vi "Stoerungen (1-64) - Anlagengrenzw..vi"(8 "Fehler (Eingang)":errorcluster caption="Fehler (Eingang, kein Fehler)") -> (0 "Fehler (Ausgang)":errorcluster)   [LabVIEW 2020, in "Stoermeldungen.lvlib"]
uses:
  Stoermeldungen.lvlib
  Stoerungen 1-64.ctl
  Seiten/Anlagengrenzwerte/Anlagen-Parameternamen.ctl
  Aktion Heizung Uebertemperatur.ctl
  Verwaltung/FGV IN Aktionen.ctl
  FGV Stoerungen Aktionen.ctl
  Aktion Anlagengrenzen pruefen.ctl
  Seiten/Anlagengrenzwerte/Anlagengrenzwerte.lvlib
  Verwaltung/Verwaltung - cRIO.lvlib
panel:
  # "Störmeldungen:\n\nAnlagengrenzwerte (1-64)"
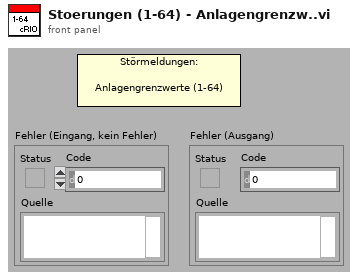
[diagram p1: front panel]
types:
  T1 = typedef "Anlagengrenzwerte.lvlib/Anlagen-Parameternamen.ctl" = enum16{"Eingangsdruck FT-IR:", "Durchfluss FT-IR:", "Durchfluss CalGas", "Druck Ausgang", "Druck Kalter Block", "Heizleitung intern", "Heizleitung zu FT-IR", "Heizung Filter:", "Heizung Pumpe:", "HL Extern SP1", "HL Extern SP2", "FT-IR Messzelle", "Schaltschrank", "Gaskühler"}
  T2 = typedef "Stoermeldungen.lvlib/FGV Stoerungen Aktionen.ctl" = enum16{"lesen", "Störung aktiv?", "1-64", "65-128"}
  T3 = typedef "Verwaltung - cRIO.lvlib/FGV IN Aktionen.ctl" = enum16{"lesen", "DI", "AI", "Fühler Br.", "TC", "Fühler Br. TC"}
  T4 = typedef "Stoermeldungen.lvlib/Aktion Heizung Uebertemperatur.ctl" = enum16{"lesen", "prüfen", "rücksetzen"}
  T5 = typedef "Stoermeldungen.lvlib/Stoerungen 1-64.ctl" = cluster{"ERR. 1":bool, "ERR. 2":bool, "ERR. 3":bool, "ERR. 4":bool, "ERR. 5":bool, "ERR. 6":bool, "ERR. 7":bool, "ERR. 8":bool, "ERR. 9":bool, "ERR. 10":bool, "ERR. 11":bool, "ERR. 12":bool, "ERR. 13":bool, "ERR. 14":bool, "ERR. 15":bool, "ERR. 16":bool, "ERR. 17":bool, "ERR. 18":bool, "ERR. 19":bool, "ERR. 20":bool, "ERR. 21":bool, "ERR. 22":bool, "ERR. 23":bool, "ERR. 24":bool, "ERR. 25":bool, "ERR. 26":bool, "ERR. 27":bool, "ERR. 28":bool, "ERR. 29":bool, "ERR. 30":bool, "ERR. 31":bool, "ERR. 32":bool, "ERR. 33":bool, "ERR. 34":bool, "ERR. 35":bool, "ERR. 36":bool, "ERR. 37":bool, "ERR. 38":bool, "ERR. 39":bool, "ERR. 40":bool, "ERR. 41":bool, "ERR. 42":bool, "ERR. 43":bool, "ERR. 44":bool, "ERR. 45":bool, "ERR. 46":bool, "ERR. 47":bool, "ERR. 48":bool, "ERR. 49":bool, "ERR. 50":bool, "ERR. 51":bool, "ERR. 52":bool, "ERR. 53":bool, "ERR. 54":bool, "ERR. 55":bool, "ERR. 56":bool, "ERR. 57":bool, "ERR. 58":bool, "ERR. 59":bool, "ERR. 60":bool, "ERR. 61":bool, "ERR. 62":bool, "ERR. 63":bool, "ERR. 64":bool}
  T6 = typedef "Verwaltung - cRIO.lvlib/TC Eingaenge.ctl" = cluster{"TC0: Reserve":sgl, "TC1: HL zu FT-IR":sgl, "TC2: HL Extern SP1":sgl, "TC3: HL Extern SP2":sgl, "TC4: Reserve":sgl, "TC5: Reserve":sgl, "TC6: Reserve":sgl, "TC7: Reserve":sgl, "TC8: FT-IR":sgl, "TC9: Reserve":sgl, "TC10: Schaltschrank":sgl, "TC11: Umgebung":sgl}
  T7 = typedef "Stoermeldungen.lvlib/Aktion Anlagengrenzen pruefen.ctl" = enum16{"Temp.", "HKL", "Druck", "SS Temp."}
  T8 = typedef "Anlagengrenzwerte.lvlib/Anlagen-Parameternamen.ctl" = enum16{"Eingangsdruck FT-IR:", "Durchfluss FT-IR:", "Druck Ausgang", "Druck Kalter Block", "Heizleitung intern", "Heizung Filter:", "Heizung Pumpe:", "HL Extern SP1", "HL Extern SP2", "FT-IR Messzelle", "Schaltschrank", "Gaskühler", "Reserve", "Flussregler"}
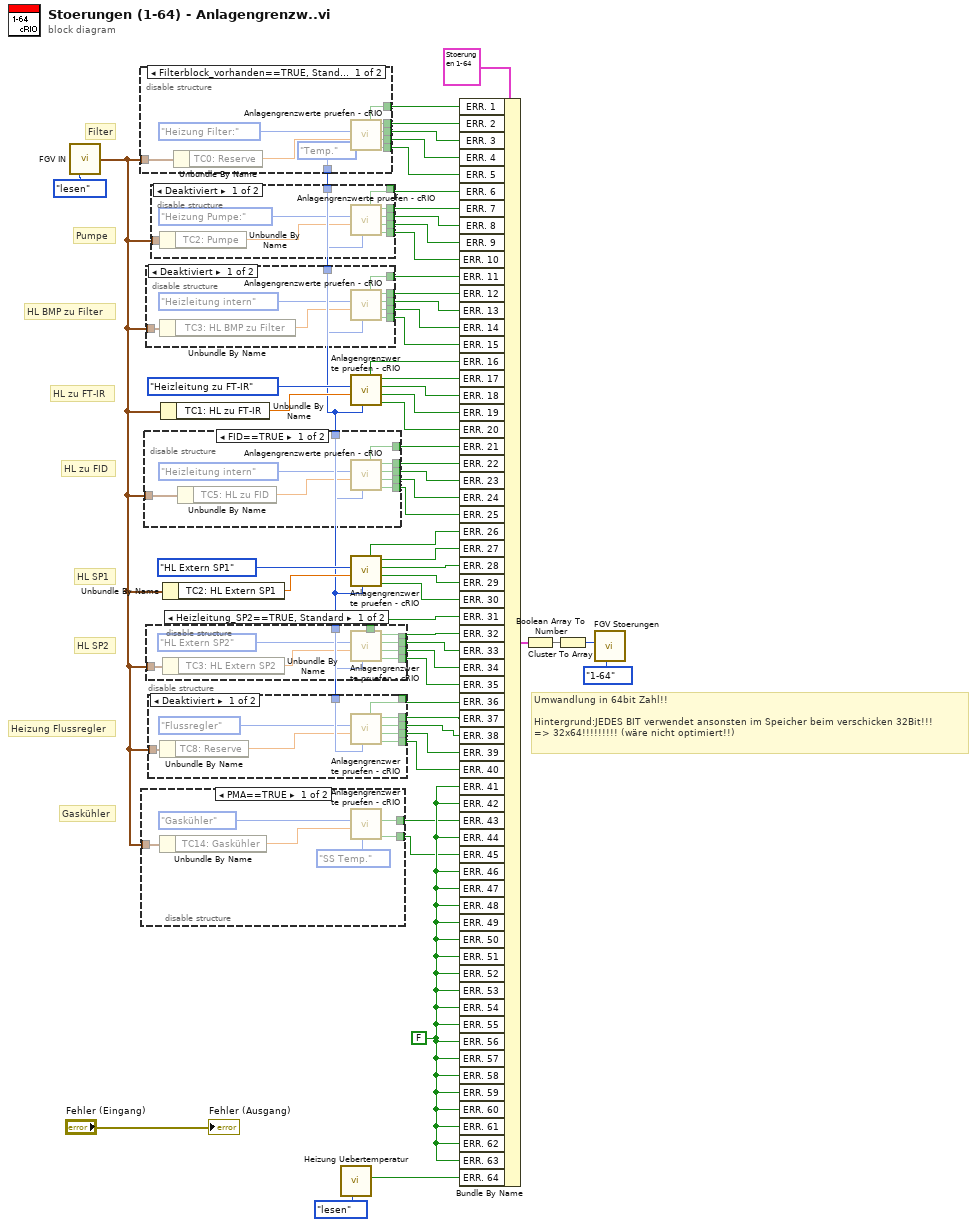
[diagram p0: block diagram]
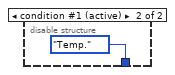
[diagram p3: hidden frame]
diagram:
  w15 = FALSE ("ERR. 52")
  # "Gaskühler"
  # "Heizung Flussregler"
  # "HL SP2"
  # "HL SP1"
  # "HL zu FT-IR"
  # "HL BMP zu Filter"
  # "HL zu FID"
  # "Pumpe"
  # "Umwandlung in 64bit Zahl!!\n\nHintergrund:JEDES BIT verwendet ansonsten im Speicher beim verschicken 32Bit!!! \n=> 32x64!!!!!!!!! (wäre nicht optimiert!!)"
  # "Filter"
  n1 = call "FGV IN.vi"("Aktion"=FGV_IN_Aktionen."lesen") -> ("TC Eingänge"=w1:T6)  [unwired: 10 in, 4 out]
  n2 = disable-structure shown="Filterblock_vorhanden==TRUE, Standard" {
    disable-tunnel: [w67 _] -> w51
    disable-tunnel: [w66 _] -> w50
    disable-tunnel: [w65 _] -> w49
    disable-tunnel: [w64 _] -> w48
    disable-tunnel: [w63 _] -> w47
    disable-tunnel: [w62 Aktion_Anlagengrenzen_pruefen."Temp." ("Aktion")] -> w4
    disable-tunnel: w1 -> [w61 _]
    frame condition #0 {
      w62 = Aktion_Anlagengrenzen_pruefen."Temp." ("Aktion")
      n3 = Unbundle By Name(w61) -> ("TC0: Reserve"=w60:sgl)
      n4 = call "Anlagengrenzwerte pruefen - cRIO.vi"("Aktion"=w62, "Wert"=w60, "Anlagen-Parametername"=Anlagen-Parameternamen."Heizung Filter:") -> ("AbschMax"=w63:bool, "AbschMin"=w64:bool, "WarnMax"=w65:bool, "WarnMin"=w66:bool, "F.Br."=w67:bool)  [unwired: 4 in]
    }
    frame condition #1 (active) {
    }
  }
  n5 = disable-structure shown="PMA==TRUE" {
    disable-tunnel: [w71 _] -> w3
    disable-tunnel: [w70 _] -> w2
    disable-tunnel: w1 -> [w69 _]
    frame condition #0 {
      n6 = Unbundle By Name(w69) -> ("TC14: Gaskühler"=w74:sgl)
      n7 = call "Anlagengrenzwerte pruefen - cRIO.vi"("Aktion"=Aktion_Anlagengrenzen_pruefen."SS Temp.", "Wert"=w74, "Anlagen-Parametername"=Anlagen-Parameternamen."Gaskühler") -> ("AbschMax"=w70:bool, "WarnMax"=w71:bool)  [unwired: 4 in, 3 out]
    }
    frame condition #1 (active) {
    }
  }
  n8 = disable-structure shown="FID==TRUE" {
    disable-tunnel: [w81 _] -> w31
    disable-tunnel: [w80 _] -> w30
    disable-tunnel: [w79 _] -> w29
    disable-tunnel: [w78 _] -> w28
    disable-tunnel: [w77 _] -> w27
    disable-tunnel: w4 -> [w76 _]
    disable-tunnel: w1 -> [w75 _]
    frame condition #0 {
      n9 = Unbundle By Name(w75) -> ("TC5: HL zu FID"=w83:sgl)
      n10 = call "Anlagengrenzwerte pruefen - cRIO.vi"("Aktion"=w76, "Wert"=w83, "Anlagen-Parametername"=Anlagen-Parameternamen."Heizleitung intern") -> ("AbschMax"=w79:bool, "AbschMin"=w78:bool, "WarnMax"=w77:bool, "WarnMin"=w80:bool, "F.Br."=w81:bool)  [unwired: 4 in]
    }
    frame condition #1 (active) {
    }
  }
  n11 = disable-structure shown="Deaktiviert" {
    disable-tunnel: [w90 _] -> w41
    disable-tunnel: [w89 _] -> w40
    disable-tunnel: [w88 _] -> w39
    disable-tunnel: [w87 _] -> w38
    disable-tunnel: [w86 _] -> w37
    disable-tunnel: w4 -> [w85 _]
    disable-tunnel: w1 -> [w84 _]
    frame Disabled {
      n12 = Unbundle By Name(w84) -> ("TC3: HL BMP zu Filter"=w92:sgl)
      n13 = call "Anlagengrenzwerte pruefen - cRIO.vi"("Aktion"=w85, "Wert"=w92, "Anlagen-Parametername"=Anlagen-Parameternamen."Heizleitung intern") -> ("AbschMax"=w88:bool, "AbschMin"=w87:bool, "WarnMax"=w86:bool, "WarnMin"=w89:bool, "F.Br."=w90:bool)  [unwired: 4 in]
    }
    frame Enabled {
    }
  }
  n14 = disable-structure shown="Heizleitung_SP2==TRUE, Standard" {
    disable-tunnel: [w101 _] -> w20
    disable-tunnel: [w100 _] -> w19
    disable-tunnel: [w99 _] -> w18
    disable-tunnel: [w98 _] -> w17
    disable-tunnel: [w97 _] -> w16
    disable-tunnel: w4 -> [w96 _]
    disable-tunnel: w1 -> [w95 _]
    frame condition #0 {
      n15 = Unbundle By Name(w95) -> ("TC3: HL Extern SP2"=w94:sgl)
      n16 = call "Anlagengrenzwerte pruefen - cRIO.vi"("Aktion"=w96, "Wert"=w94, "Anlagen-Parametername"=Anlagen-Parameternamen."HL Extern SP2") -> ("AbschMax"=w97:bool, "AbschMin"=w98:bool, "WarnMax"=w99:bool, "WarnMin"=w100:bool, "F.Br."=w101:bool)  [unwired: 4 in]
    }
    frame condition #1 (active) {
    }
  }
  n17 = disable-structure shown="Deaktiviert" {
    disable-tunnel: [w110 _] -> w9
    disable-tunnel: [w109 _] -> w8
    disable-tunnel: [w108 _] -> w7
    disable-tunnel: [w107 _] -> w6
    disable-tunnel: [w106 _] -> w5
    disable-tunnel: w4 -> [w105 _]
    disable-tunnel: w1 -> [w104 _]
    frame Disabled {
      n18 = Unbundle By Name(w104) -> ("TC8: Reserve"=w102:sgl)
      n19 = call "Anlagengrenzwerte pruefen - cRIO.vi"("Aktion"=w105, "Wert"=w102, "Anlagen-Parametername"=Anlagen-Parameternamen."Flussregler") -> ("AbschMax"=w106:bool, "AbschMin"=w107:bool, "WarnMax"=w108:bool, "WarnMin"=w109:bool, "F.Br."=w110:bool)  [unwired: 4 in]
    }
    frame Enabled {
    }
  }
  n20 = disable-structure shown="Deaktiviert" {
    disable-tunnel: [w119 _] -> w46
    disable-tunnel: [w118 _] -> w45
    disable-tunnel: [w117 _] -> w44
    disable-tunnel: [w116 _] -> w43
    disable-tunnel: [w115 _] -> w42
    disable-tunnel: w4 -> [w114 _]
    disable-tunnel: w1 -> [w113 _]
    frame Disabled {
      n21 = Unbundle By Name(w113) -> ("TC2: Pumpe"=w112:sgl)
      n22 = call "Anlagengrenzwerte pruefen - cRIO.vi"("Aktion"=w114, "Wert"=w112, "Anlagen-Parametername"=Anlagen-Parameternamen."Heizung Pumpe:") -> ("AbschMax"=w116:bool, "AbschMin"=w115:bool, "WarnMax"=w117:bool, "WarnMin"=w118:bool, "F.Br."=w119:bool)  [unwired: 4 in]
    }
    frame Enabled {
    }
  }
  n23 = Unbundle By Name(w1) -> ("TC1: HL zu FT-IR"=w54:sgl)
  n24 = Unbundle By Name(w1) -> ("TC2: HL Extern SP1"=w10:sgl)
  n25 = call "Heizung Uebertemperatur.vi"("Aktionen"=Aktion_Heizung_Uebertemperatur."lesen") -> ("Heizung Übertemperatur"=w26:bool)  [unwired: 9 in, 1 out]
  n26 = call "Anlagengrenzwerte pruefen - cRIO.vi"("Aktion"=w4, "Wert"=w54, "Anlagen-Parametername"=Anlagen-Parameternamen."Heizleitung zu FT-IR") -> ("AbschMax"=w34:bool, "AbschMin"=w33:bool, "WarnMax"=w32:bool, "WarnMin"=w36:bool, "F.Br."=w35:bool)  [unwired: 4 in]
  n27 = call "Anlagengrenzwerte pruefen - cRIO.vi"("Aktion"=w4, "Wert"=w10, "Anlagen-Parametername"=Anlagen-Parameternamen."HL Extern SP1") -> ("AbschMax"=w21:bool, "AbschMin"=w22:bool, "WarnMax"=w23:bool, "WarnMin"=w24:bool, "F.Br."=w25:bool)  [unwired: 4 in]
  n28 = Bundle By Name(cluster=T5 {"ERR. 1"=FALSE, "ERR. 2"=FALSE, "ERR. 3"=FALSE, "ERR. 4"=FALSE, "ERR. 5"=FALSE, "ERR. 6"=FALSE, "ERR. 7"=FALSE, "ERR. 8"=FALSE, "ERR. 9"=FALSE, "ERR. 10"=FALSE, "ERR. 11"=FALSE, "ERR. 12"=FALSE, "ERR. 13"=FALSE, "ERR. 14"=FALSE, "ERR. 15"=FALSE, "ERR. 16"=FALSE, "ERR. 17"=FALSE, "ERR. 18"=FALSE, "ERR. 19"=FALSE, "ERR. 20"=FALSE, "ERR. 21"=FALSE, "ERR. 22"=FALSE, "ERR. 23"=FALSE, "ERR. 24"=FALSE, "ERR. 25"=FALSE, "ERR. 26"=FALSE, "ERR. 27"=FALSE, "ERR. 28"=FALSE, "ERR. 29"=FALSE, "ERR. 30"=FALSE, "ERR. 31"=FALSE, "ERR. 32"=FALSE, "ERR. 33"=FALSE, "ERR. 34"=FALSE, "ERR. 35"=FALSE, "ERR. 36"=FALSE, "ERR. 37"=FALSE, "ERR. 38"=FALSE, "ERR. 39"=FALSE, "ERR. 40"=FALSE, "ERR. 41"=FALSE, "ERR. 42"=FALSE, "ERR. 43"=FALSE, "ERR. 44"=FALSE, "ERR. 45"=FALSE, "ERR. 46"=FALSE, "ERR. 47"=FALSE, "ERR. 48"=FALSE, "ERR. 49"=FALSE, "ERR. 50"=FALSE, "ERR. 51"=FALSE, "ERR. 52"=FALSE, "ERR. 53"=FALSE, "ERR. 54"=FALSE, "ERR. 55"=FALSE, "ERR. 56"=FALSE, "ERR. 57"=FALSE, "ERR. 58"=FALSE, "ERR. 59"=FALSE, "ERR. 60"=FALSE, "ERR. 61"=FALSE, "ERR. 62"=FALSE, "ERR. 63"=FALSE, "ERR. 64"=FALSE} ("STÖRUNGEN"), "ERR. 1"=w51, "ERR. 2"=w50, "ERR. 3"=w49, "ERR. 4"=w48, "ERR. 5"=w47, "ERR. 6"=w46, "ERR. 7"=w45, "ERR. 8"=w44, "ERR. 9"=w42, "ERR. 10"=w43, "ERR. 11"=w41, "ERR. 12"=w40, "ERR. 13"=w37, "ERR. 14"=w38, "ERR. 15"=w39, "ERR. 16"=w35, "ERR. 17"=w36, "ERR. 18"=w32, "ERR. 19"=w33, "ERR. 20"=w34, "ERR. 21"=w31, "ERR. 22"=w30, "ERR. 23"=w27, "ERR. 24"=w28, "ERR. 25"=w29, "ERR. 26"=w25, "ERR. 27"=w24, "ERR. 28"=w23, "ERR. 29"=w22, "ERR. 30"=w21, "ERR. 31"=w20, "ERR. 32"=w19, "ERR. 33"=w18, "ERR. 34"=w17, "ERR. 35"=w16, "ERR. 36"=w9, "ERR. 37"=w8, "ERR. 38"=w7, "ERR. 39"=w6, "ERR. 40"=w5, "ERR. 41"=w15, "ERR. 42"=w15, "ERR. 43"=w3, "ERR. 44"=w15, "ERR. 45"=w2, "ERR. 46"=w15, "ERR. 47"=w15, "ERR. 48"=w15, "ERR. 49"=w15, "ERR. 50"=w15, "ERR. 51"=w15, "ERR. 52"=w15, "ERR. 53"=w15, "ERR. 54"=w15, "ERR. 55"=w15, "ERR. 56"=w15, "ERR. 57"=w15, "ERR. 58"=w15, "ERR. 59"=w15, "ERR. 60"=w15, "ERR. 61"=w15, "ERR. 62"=w15, "ERR. 63"=w15, "ERR. 64"=w26) -> (w56:T5)
  n29 = Cluster To Array(cluster=w56) -> (array=w55:bool[])
  n30 = Boolean Array To Number ("Boolesches Array nach Zahl")(Boolean array=w55) -> (number=w12:u64)
  n31 = call "FGV Stoerungen.vi"("Aktionen"=FGV_Stoerungen_Aktionen."1-64", "1-64"=w12) -> ()  [unwired: 7 in, 3 out]
  "Fehler (Ausgang)" <- "Fehler (Eingang)"
